vi "testSpeedAngles.vi"() -> ()   [LabVIEW 2015]
uses:
  ARM angles.vi
panel:
  out "q2":i32
  out "q1":i32
  in  "stop 2":bool
  in  "elbow speed":i16
  in  "elbow angle":i32(slide) scale=-90.0..90.0
  in  "shoulder speed":i16
  in  "shoulder angle":i32(slide) scale=-30.0..40.0
  in  "stop":bool
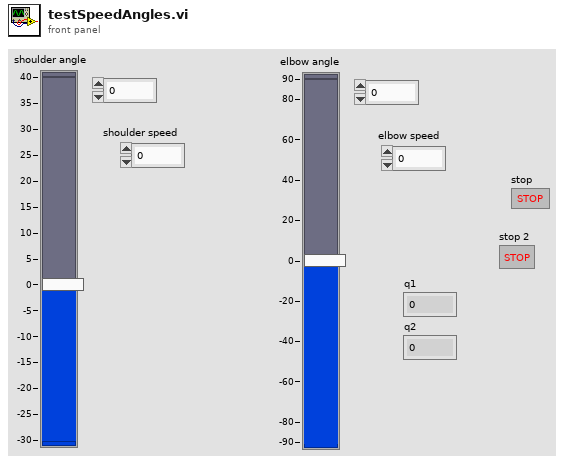
[diagram p1: front panel]
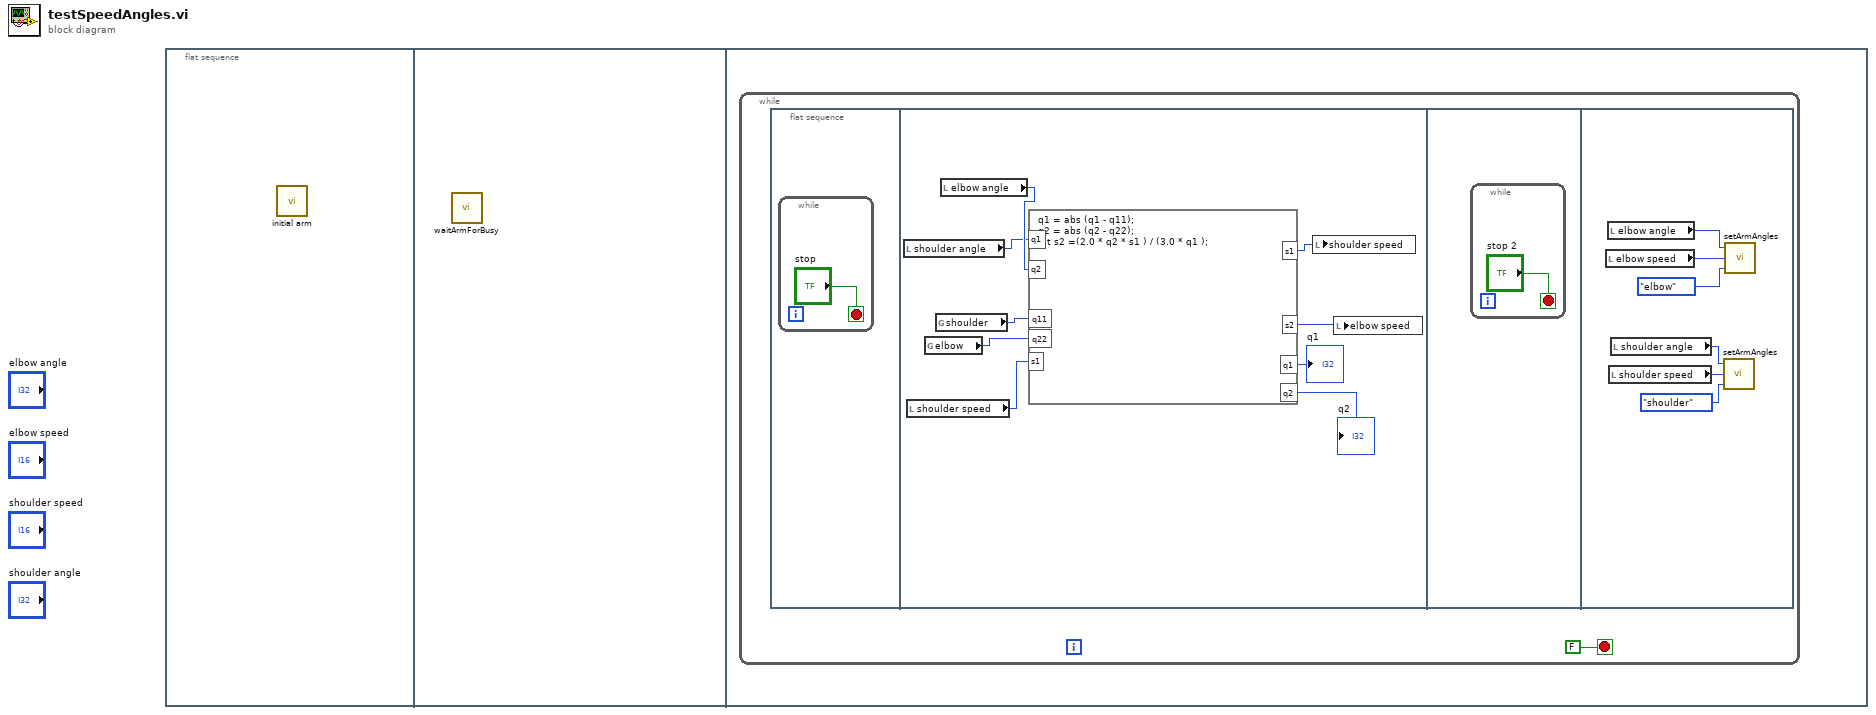
[diagram p0: block diagram]
diagram:
  n1 = flat-sequence {
    frame #0 {
      n2 = call "initial arm.vi"() -> ()  [unwired: 12 in]
    }
    frame #1 {
      n3 = call "waitArmForBusy.vi"() -> ()  [unwired: 12 in]
    }
    frame #2 {
      n4 = while {
        stop <- FALSE stop-if-true
        n5 = flat-sequence {
          frame #0 {
            n6 = while {
              stop <- "stop" stop-if-true
            }
          }
          frame #1 {
            n7 = local read "shoulder angle"() -> (w8:i32)
            n8 = local read "shoulder speed"() -> (w7:i16)
            n9 = global read "ARM angles.vi" "elbow"() -> (w10:i32)
            n10 = global read "ARM angles.vi" "shoulder"() -> (w11:i32)
            n11 = local read "elbow angle"() -> (w9:i32)
            n12 = formula code="q1 = abs (q1 - q11);\nq2 = abs (q2 - q22);\nint s2 =(2.0 * q2 * s1 ) / (3.0 * q1 );"("q1"=w8, "q2"=w9, "s1"=w7, "q11"=w11, "q22"=w10) -> ("s1"=w6:i16, "s2"=w5:i32, "q1"=→"q1":i32, "q2"=→"q2":i32)
            n13 = local write "shoulder speed"(w6) -> ()
            n14 = local write "elbow speed"(w5) -> ()
          }
          frame #2 {
            n15 = while {
              stop <- "stop 2" stop-if-true
            }
          }
          frame #3 {
            n16 = local read "elbow speed"() -> (w17:i16)
            n17 = local read "elbow angle"() -> (w16:i32)
            n18 = local read "shoulder speed"() -> (w14:i16)
            n19 = local read "shoulder angle"() -> (w13:i32)
            n20 = call "setArmAngles.vi"("Enum"=enum16{"shoulder", "elbow"}."shoulder", "speed"=w14, "angle"=w13) -> ()  [unwired: 1 in]
            n21 = call "setArmAngles.vi"("Enum"=enum16{"shoulder", "elbow"}."elbow", "speed"=w17, "angle"=w16) -> ()  [unwired: 1 in]
          }
        }
      }
    }
  }
